vi "Init_KCubeDCServo.vi"(10 "SerialNumber":string="27251750", 11 ".NET Refnum in":refnum<k24>(container)) -> (1 "get paras Cluster":T1, 2 "Device":refnum<k24>, 3 ".NET Refnum out":refnum<k24>)   [LabVIEW 2019]
doc: "init and set low-level parameters to dc servo motor"
uses:
  D:/Victor Sun/optical trap control/Kinesis/Thorlabs.MotionControl.Controls.dll
  Kinesis/Thorlabs.MotionControl.Controls.dll
  D:/Victor Sun/optical trap control/Kinesis/ThorLabs.MotionControl.KCube.DCServoCLI.dll
  Kinesis/ThorLabs.MotionControl.KCube.DCServoCLI.dll
  D:/Victor Sun/optical trap control/Kinesis/Thorlabs.MotionControl.GenericMotorCLI.dll
  Kinesis/Thorlabs.MotionControl.GenericMotorCLI.dll
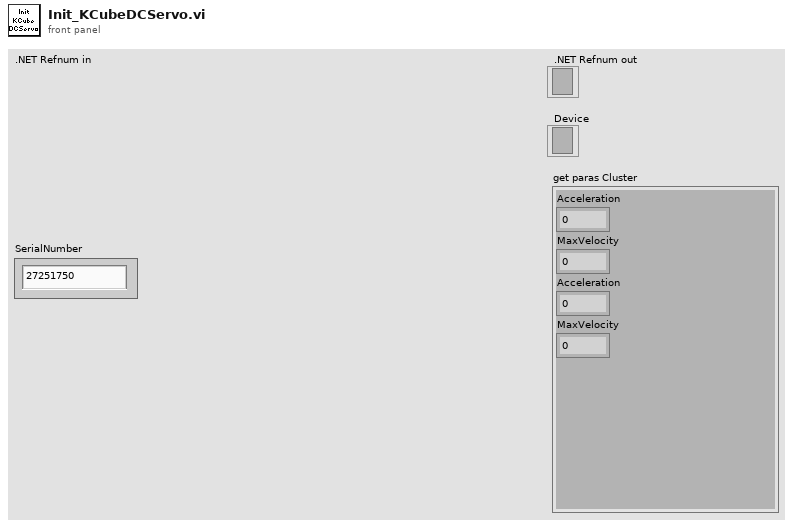
[diagram p1: front panel]
types:
  T1 = cluster{"Acceleration":dbl, "MaxVelocity":dbl, "Acceleration":dbl, "MaxVelocity":dbl}
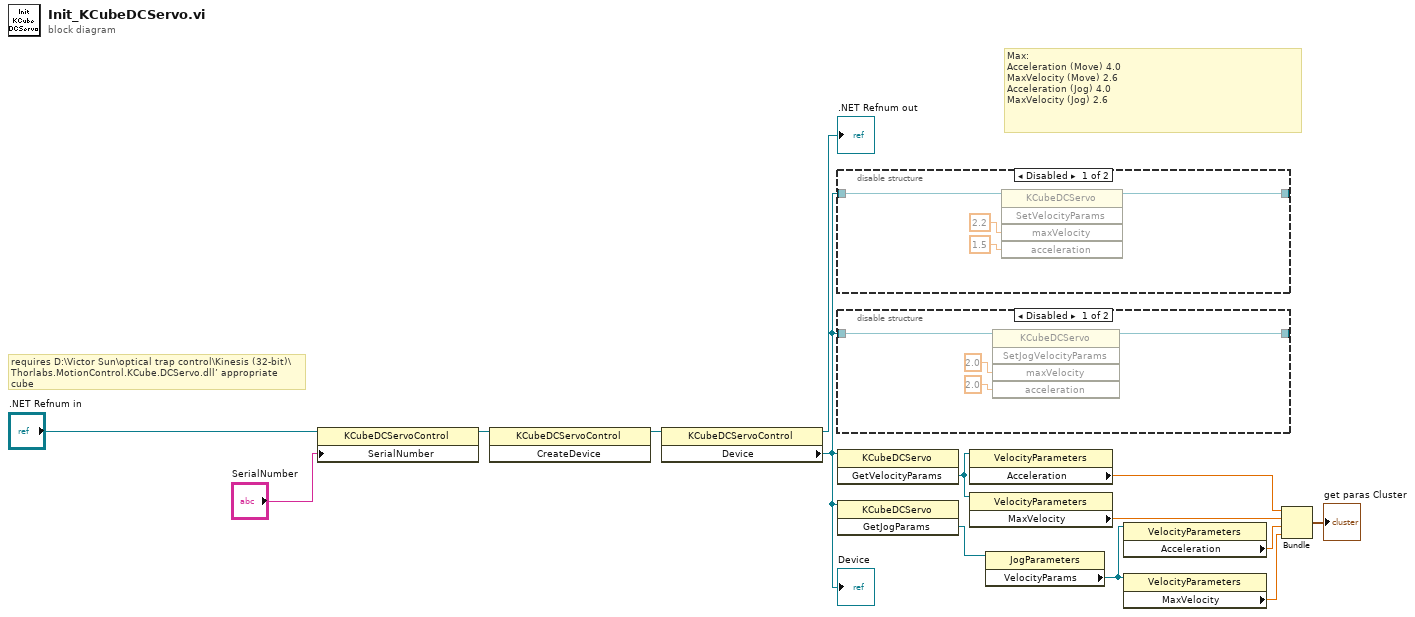
[diagram p0: block diagram]
diagram:
  # "Max:\nAcceleration (Move) 4.0\nMaxVelocity (Move) 2.6\nAcceleration (Jog) 4.0\nMaxVelocity (Jog) 2.6"
  # "requires D:\\Victor Sun\\optical trap control\\Kinesis (32-bit)\\Thorlabs.MotionControl.KCube.DCServo.dll’ appropriate cube"
  n1 = property class="KCubeDCServoControl"(reference=".NET Refnum in", "SerialNumber"="SerialNumber") -> (reference out=w3:refnum<k24>)  [unwired: 1 in, 1 out]
  n2 = invoke class="KCubeDCServoControl" method="CreateDevice"(reference=w3) -> (reference out=w9:refnum<k24>)  [unwired: 2 in, 2 out]
  n3 = property class="KCubeDCServoControl"(reference=w9) -> (reference out=→".NET Refnum out":refnum<k24>, "Device"=w8:refnum<k24>)  [unwired: 1 in, 1 out]
  "Device" <- w8
  n4 = disable-structure shown="Disabled" {
    disable-tunnel: [w16 _] -> _
    disable-tunnel: w8 -> [w15 _]
    frame Disabled {
      n5 = invoke class="KCubeDCServo" method="SetVelocityParams"(reference=w15, "maxVelocity"=2.2, "acceleration"=1.5) -> (reference out=w16:refnum<k24>)  [unwired: 2 in, 4 out]
    }
    frame Enabled {
    }
  }
  n6 = disable-structure shown="Disabled" {
    disable-tunnel: [w20 _] -> _
    disable-tunnel: w8 -> [w19 _]
    frame Disabled {
      n7 = invoke class="KCubeDCServo" method="SetJogVelocityParams"(reference=w19, "maxVelocity"=2.0, "acceleration"=2.0) -> (reference out=w20:refnum<k24>)  [unwired: 2 in, 4 out]
    }
    frame Enabled {
    }
  }
  n8 = invoke class="KCubeDCServo" method="GetVelocityParams"(reference=w8) -> ("GetVelocityParams"=w7:refnum<k24>)  [unwired: 2 in, 2 out]
  n9 = invoke class="KCubeDCServo" method="GetJogParams"(reference=w8) -> ("GetJogParams"=w5:refnum<k24>)  [unwired: 2 in, 2 out]
  n10 = property class="VelocityParameters"(reference=w7) -> ("Acceleration"=w11:dbl)  [unwired: 1 in, 2 out]
  n11 = property class="VelocityParameters"(reference=w7) -> ("MaxVelocity"=w12:dbl)  [unwired: 1 in, 2 out]
  n12 = property class="JogParameters"(reference=w5) -> ("VelocityParams"=w6:refnum<k24>)  [unwired: 1 in, 2 out]
  n13 = property class="VelocityParameters"(reference=w6) -> ("Acceleration"=w13:dbl)  [unwired: 1 in, 2 out]
  n14 = property class="VelocityParameters"(reference=w6) -> ("MaxVelocity"=w14:dbl)  [unwired: 1 in, 2 out]
  n15 = Bundle("Acceleration"=w11, "MaxVelocity"=w12, "Acceleration"=w13, "MaxVelocity"=w14) -> (→"get paras Cluster":T1)  [unwired: 1 in]
